vi "LSMcontroller_v56_from here for labview64bit.vi"() -> ()   [LabVIEW 2015] (continued)
                n3094 = property on="square matrix" class="Bool (strict)"("Value"=TRUE ("square matrix")) -> ()  [unwired: 2 in, 2 out]
                n3095 = property on="Square pixels" class="Bool (strict)"("Value"=FALSE ("square matrix")) -> ()  [unwired: 2 in, 2 out]
              }
            }
          }
          event "up", "downright", "down", "downleft", "right", "left", "upright", "upleft": Value Change {
            n3096 = event-data() -> ()  [unwired: 1 in, 6 out]
            n3097 = local read "downright"() -> (w6201:bool)
            n3098 = local read "downleft"() -> (w6203:bool)
            n3099 = local read "upright"() -> (w6199:bool)
            n3100 = local read "upleft"() -> (w6197:bool)
            n3101 = local read "down"() -> (w6202:bool)
            n3102 = local read "right"() -> (w6200:bool)
            n3103 = local read "left"() -> (w6204:bool)
            n3104 = local read "up"() -> (w6198:bool)
            n3105 = Compound Arithmetic op=OR(w6197, w6198, w6199, w6200, w6201, w6202, w6203, w6204) -> (w6196:bool)
            n3106 = case shown="True" w6196 {
              frame False {
              }
              frame True {
                n3107 = stacked-sequence {
                  frame #0 {
                    n3108 = local read "downright"() -> (w6206:bool)
                    n3109 = local read "downleft"() -> (w6208:bool)
                    n3110 = local read "BigSmall"() -> (w6205:bool)
                    n3111 = local read "upright"() -> (w6210:bool)
                    n3112 = local read "upleft"() -> (w6213:bool)
                    n3113 = local read "down"() -> (w6209:bool)
                    n3114 = local read "right"() -> (w6211:bool)
                    n3115 = local read "left"() -> (w6207:bool)
                    n3116 = local read "up"() -> (w6212:bool)
                    n3117 = call "movestageparams.vi"("command"="get") -> ("Params out"=w6216:T22)  [unwired: 1 in]
                    n3118 = Bundle By Name(cluster=w6216, "upleft"=w6213, "up"=w6212, "upright"=w6210, "right"=w6211, "downright"=w6206, "down"=w6209, "downleft"=w6208, "left"=w6207, "Bigsmall"=w6205) -> (w6217:T22)
                    n3119 = call "movestageparams.vi"("Params in"=w6217, "command"="set") -> ()  [unwired: 1 out]
                  }
                  frame #1 {
                    n3120 = disable-structure shown="Disabled" {
                      frame Disabled {
                        n3121 = call "configuration.vi"("command"="get") -> ("config out"=w6220:T13)  [unwired: 2 in, 1 out]
                        n3122 = in-place {
                          n3123 = in-place-cluster #45(w6220) -> ()  [unwired: 2 out]
                          n3124 = in-place-cluster #45("StageL"="StageL", "StageS"="StageS") -> (w6218:T13)
                        }
                        n3125 = call "configuration.vi"("config in"=w6218, "command"="set") -> ()  [unwired: 1 in, 2 out]
                      }
                      frame Enabled {
                      }
                    }
                  }
                  frame #2 {
                    n3126 = call "movestage.vi"() -> ()  [unwired: 12 in]
                  }
                  frame #3 {
                    w6224 = FALSE ("OK Button")
                    w6225 = FALSE ("OK Button")
                    n3127 = property on="down" class="Bool (strict)"("Value"=w6225) -> ()  [unwired: 2 in, 2 out]
                    n3128 = property on="up" class="Bool (strict)"("Value"=w6225) -> ()  [unwired: 2 in, 2 out]
                    n3129 = property on="right" class="Bool (strict)"("Value"=w6225) -> ()  [unwired: 2 in, 2 out]
                    n3130 = property on="left" class="Bool (strict)"("Value"=w6225) -> ()  [unwired: 2 in, 2 out]
                    n3131 = property on="upright" class="Bool (strict)"("Value"=w6224) -> ()  [unwired: 2 in, 2 out]
                    n3132 = property on="downleft" class="Bool (strict)"("Value"=w6224) -> ()  [unwired: 2 in, 2 out]
                    n3133 = property on="downright" class="Bool (strict)"("Value"=w6224) -> ()  [unwired: 2 in, 2 out]
                    n3134 = property on="upleft" class="Bool (strict)"("Value"=w6224) -> ()  [unwired: 2 in, 2 out]
                  }
                }
              }
            }
          }
          event "finite samples": Value Change {
            n3135 = event-data() -> ("NewVal"=w6226:bool)  [unwired: 1 in]
            n3136 = flat-sequence {
              tunnel: w6226 -> [w6227]
              frame #0 {
                n3137 = case shown="True" w6227 {
                  frame False {
                    w6228 = FALSE ("wavdet")
                    n3138 = property on="continuous" class="Bool (strict)"("Value"=TRUE ("continuous for display")) -> ()  [unwired: 2 in, 2 out]
                    n3139 = property on="wavdet" class="Bool (strict)"("Value"=w6228) -> ()  [unwired: 2 in, 2 out]
                    n3140 = property on="save\ndata" class="Bool (strict)"("Value"=w6228) -> ()  [unwired: 2 in, 2 out]
                    n3141 = property on="# of frames" class="DigNum (strict)"("DisabledEnum"=T8."Disabled and Grayed Out" ("Disabled")) -> ()  [unwired: 2 in, 2 out]
                    n3142 = property on="save\ndata" class="Bool (strict)"("DisabledEnum"=T8."Disabled and Grayed Out" ("Disabled")) -> ()  [unwired: 2 in, 2 out]
                    "Save tab" <- enum32{"withsave", "withoutsave"}."withsave" ("Save tab")
                  }
                  frame True {
                    w6235 = FALSE ("continuous for display")
                    n3143 = property on="continuous" class="Bool (strict)"("Value"=w6235) -> ()  [unwired: 2 in, 2 out]
                    n3144 = property on="wavdet" class="Bool (strict)"("Value"=w6235) -> ()  [unwired: 2 in, 2 out]
                    n3145 = local write "Save tab"(enum32{"withsave", "withoutsave"}."withsave" ("Save tab")) -> ()
                    n3146 = property on="save\ndata" class="Bool (strict)"("DisabledEnum"=T8."Enabled" ("Disabled")) -> ()  [unwired: 2 in, 2 out]
                    n3147 = property on="save\ndata" class="Bool (strict)"("Value"=TRUE ("save\ndata")) -> ()  [unwired: 2 in, 2 out]
                    n3148 = property on="# of frames" class="DigNum (strict)"("DisabledEnum"=T8."Enabled" ("Disabled")) -> ()  [unwired: 2 in, 2 out]
                  }
                }
              }
              frame #1 {
                n3149 = local read "finite samples"() -> (w6244:bool)
                n3150 = local read "continuous"() -> (w6243:bool)
                n3151 = local read "wavdet"() -> (w6242:bool)
                n3152 = call "2pparameters.vi"("command"="get") -> ("params out"=w6238:T12)  [unwired: 1 in]
                n3153 = Bundle By Name(cluster=w6238, "finite"=w6244, "cont"=w6243, "wavdet"=w6242) -> (w6241:T12)
                n3154 = call "2pparameters.vi"("Params in"=w6241, "command"="set") -> ()  [unwired: 1 out]
              }
            }
          }
          event "continuous": Value Change {
            n3155 = event-data() -> ("NewVal"=w6245:bool)  [unwired: 1 in]
            n3156 = flat-sequence {
              tunnel: w6245 -> [w6246]
              frame #0 {
                n3157 = case shown="True" w6246 {
                  frame False {
                    n3158 = property on="finite samples" class="Bool (strict)"("Value"=TRUE ("finite samples for recording")) -> ()  [unwired: 2 in, 2 out]
                    n3159 = property on="save\ndata" class="Bool (strict)"("Value"=TRUE ("save\ndata")) -> ()  [unwired: 2 in, 2 out]
                    n3160 = property on="wavdet" class="Bool (strict)"("Value"=FALSE ("wavdet")) -> ()  [unwired: 2 in, 2 out]
                    n3161 = local write "Save tab"(enum32{"withsave", "withoutsave"}."withsave" ("Save tab")) -> ()
                    n3162 = property on="# of frames" class="DigNum (strict)"("DisabledEnum"=T8."Enabled" ("Disabled")) -> ()  [unwired: 2 in, 2 out]
                    n3163 = property on="save\ndata" class="Bool (strict)"("DisabledEnum"=T8."Enabled" ("Disabled")) -> ()  [unwired: 2 in, 2 out]
                  }
                  frame True {
                    w6253 = FALSE ("finite samples for recording")
                    n3164 = property on="finite samples" class="Bool (strict)"("Value"=w6253) -> ()  [unwired: 2 in, 2 out]
                    n3165 = property on="wavdet" class="Bool (strict)"("Value"=w6253) -> ()  [unwired: 2 in, 2 out]
                    n3166 = property on="save\ndata" class="Bool (strict)"("Value"=w6253) -> ()  [unwired: 2 in, 2 out]
                    n3167 = local write "Save tab"(enum32{"withsave", "withoutsave"}."withsave" ("Save tab")) -> ()
                    n3168 = property on="# of frames" class="DigNum (strict)"("DisabledEnum"=T8."Disabled and Grayed Out" ("Disabled")) -> ()  [unwired: 2 in, 2 out]
                    n3169 = property on="save\ndata" class="Bool (strict)"("DisabledEnum"=T8."Disabled and Grayed Out" ("Disabled")) -> ()  [unwired: 2 in, 2 out]
                  }
                }
              }
              frame #1 {
                n3170 = local read "finite samples"() -> (w6263:bool)
                n3171 = local read "continuous"() -> (w6262:bool)
                n3172 = local read "wavdet"() -> (w6261:bool)
                n3173 = call "2pparameters.vi"("command"="get") -> ("params out"=w6257:T12)  [unwired: 1 in]
                n3174 = Bundle By Name(cluster=w6257, "finite"=w6263, "cont"=w6262, "wavdet"=w6261) -> (w6260:T12)
                n3175 = call "2pparameters.vi"("Params in"=w6260, "command"="set") -> ()  [unwired: 1 out]
              }
            }
          }
          event "wavdet": Value Change {
            n3176 = event-data() -> ("NewVal"=w6264:bool)  [unwired: 1 in]
            n3177 = flat-sequence {
              tunnel: w6264 -> [w6265]
              frame #0 {
                n3178 = case shown="False" w6265 {
                  frame False {
                    n3179 = property on="finite samples" class="Bool (strict)"("Value"=TRUE ("finite samples for recording")) -> ()  [unwired: 2 in, 2 out]
                    n3180 = property on="continuous" class="Bool (strict)"("Value"=FALSE ("continuous")) -> ()  [unwired: 2 in, 2 out]
                    n3181 = local write "Save tab"(enum32{"withsave", "withoutsave"}."withsave" ("Save tab")) -> ()
                    n3182 = property on="save\ndata" class="Bool (strict)"("DisabledEnum"=T8."Enabled" ("Disabled")) -> ()  [unwired: 2 in, 2 out]
                    n3183 = property on="# of frames" class="DigNum (strict)"("DisabledEnum"=T8."Enabled" ("Disabled")) -> ()  [unwired: 2 in, 2 out]
                    n3184 = property on="save\ndata" class="Bool (strict)"("Value"=TRUE ("save\ndata")) -> ()  [unwired: 2 in, 2 out]
                  }
                  frame True {
                    w6274 = FALSE ("finite samples for recording")
                    n3185 = property on="finite samples" class="Bool (strict)"("Value"=w6274) -> ()  [unwired: 2 in, 2 out]
                    n3186 = property on="continuous" class="Bool (strict)"("Value"=w6274) -> ()  [unwired: 2 in, 2 out]
                    n3187 = property on="save\ndata" class="Bool (strict)"("DisabledEnum"=T8."Enabled" ("Disabled")) -> ()  [unwired: 2 in, 2 out]
                    n3188 = local write "Save tab"(enum32{"withsave", "withoutsave"}."withsave" ("Save tab")) -> ()
                    n3189 = property on="# of frames" class="DigNum (strict)"("DisabledEnum"=T8."Disabled" ("Disabled")) -> ()  [unwired: 2 in, 2 out]
                    n3190 = property on="save\ndata" class="Bool (strict)"("Value"=TRUE ("save\ndata")) -> ()  [unwired: 2 in, 2 out]
                  }
                }
              }
              frame #1 {
                n3191 = local read "finite samples"() -> (w6277:bool)
                n3192 = local read "continuous"() -> (w6278:bool)
                n3193 = local read "wavdet"() -> (w6279:bool)
                n3194 = call "2pparameters.vi"("command"="get") -> ("params out"=w6283:T12)  [unwired: 1 in]
                n3195 = Bundle By Name(cluster=w6283, "finite"=w6277, "cont"=w6278, "wavdet"=w6279) -> (w6280:T12)
                n3196 = call "2pparameters.vi"("Params in"=w6280, "command"="set") -> ()  [unwired: 1 out]
              }
            }
          }
          event "cursors": Value Change {
            n3197 = event-data() -> ()  [unwired: 1 in, 5 out]
            n3198 = case shown="True" "cursors" {
              frame False {
                n3199 = property on="img_CH1" class="IntGraph (strict)"("Active Cursor"=u32 0, "Cursor.Cursor Style"=u8 0 ("Cursor Style"), "Cursor.Cursor Point Style"=u8 0 ("Cursor Point Style")) -> ("Cursor.Cursor Position:Cursor X"=w6288:dbl, "Cursor.Cursor Position:Cursor Y"=w6289:dbl)  [unwired: 2 in, 2 out]
                n3200 = property on="img_CH2" class="IntGraph (strict)"("Active Cursor"=u32 0, "Cursor.Cursor Style"=u8 0 ("Cursor Style"), "Cursor.Cursor Point Style"=u8 0 ("Cursor Point Style")) -> ()  [unwired: 2 in, 2 out]
                n3201 = local write "cursor x [pixel]"(w6288) -> ()
                n3202 = local write "cursor y [pixel]"(w6289) -> ()
              }
              frame True {
                n3203 = stacked-sequence {
                  frame #0 {
                    n3204 = call "2pparameters.vi"("command"="get") -> ("params out"=w6304:T12)  [unwired: 1 in]
                    n3205 = Unbundle By Name(w6304) -> ("Xpixels Img"=w6305:i32, "Ypixels Img"=w6302:i32)
                    n3206 = To Double Precision Float(number=w6302) -> (double precision float=w6296:dbl)
                    n3207 = To Double Precision Float(number=w6305) -> (double precision float=w6301:dbl)
                    n3208 = Divide(x=w6296, y=2.0) -> (x/y=w6297:dbl)
                    n3209 = Divide(x=w6301, y=2.0) -> (x/y=w6299:dbl)
                    n3210 = Round To Nearest(number=w6297) -> (nearest integer value=w6295:dbl)
                    n3211 = Round To Nearest(number=w6299) -> (nearest integer value=w6298:dbl)
                    n3212 = property on="img_CH1" class="IntGraph (strict)"("Active Cursor"=u32 0, "Cursor.Cursor Style"=u8 8 ("Cursor Style"), "Cursor.Cursor Point Style"=u8 5 ("Cursor Point Style"), "Cursor.Cursor Position:Cursor X"=w6298, "Cursor.Cursor Position:Cursor Y"=w6295, "Cursor.Visible"=TRUE) -> ()  [unwired: 2 in, 2 out]
                  }
                  frame #1 {
                    n3213 = call "2pparameters.vi"("command"="get") -> ("params out"=w6324:T12)  [unwired: 1 in]
                    n3214 = call "2pparameters.vi"("command"="get") -> ("params out"=w6322:T12)  [unwired: 1 in]
                    n3215 = property on="img_CH1" class="IntGraph (strict)"("Active Cursor"=u32 0, "Cursor.Cursor Style"=u8 8 ("Cursor Style"), "Cursor.Cursor Point Style"=u8 5 ("Cursor Point Style")) -> ("Cursor.Cursor Position:Cursor X"=w6317:dbl, "Cursor.Cursor Position:Cursor Y"=w6316:dbl, "Cursor.Cursor Index"=w6339:i32, "Cursor.Cursor Plot"=w6338:i32, "Cursor.Visible"=w6309:bool)  [unwired: 2 in, 2 out]
                    "cursor x [pixel]" <- w6317
                    "cursor y [pixel]" <- w6316
                    n3216 = Unbundle By Name(w6324) -> ("Vy-max Img"=w6326:dbl, "Vy-min Img"=w6313:dbl, "Ypixels Img"=w6328:i32)
                    n3217 = Unbundle By Name(w6322) -> ("VX-max Img"=w6323:dbl, "Vx-min Img"=w6311:dbl, "Xpixels Img"=w6327:i32)
                    n3218 = Subtract(x=w6326, y=w6313) -> (x-y=w6331:dbl)
                    n3219 = Subtract(x=w6323, y=w6311) -> (x-y=w6329:dbl)
                    n3220 = local read "img_CH2"() -> (w6335:sgl[][])
                    n3221 = To Double Precision Float(number=w6327) -> (double precision float=w6330:dbl)
                    n3222 = local read "img_CH1"() -> (w6336:sgl[][])
                    n3223 = To Double Precision Float(number=w6328) -> (double precision float=w6332:dbl)
                    n3224 = Index Array(array=w6336, index (row)=w6339, index (col)=w6338) -> (element=→"value CH 1":sgl)
                    n3225 = Index Array(array=w6335, index (row)=w6339, index (col)=w6338) -> (element=→"value CH 2":sgl)
                    n3226 = Divide(x=w6329, y=w6330) -> (x/y=w6333:dbl)
                    n3227 = Divide(x=w6331, y=w6332) -> (x/y=w6334:dbl)
                    n3228 = Multiply(x=w6317, y=w6333) -> (x*y=w6312:dbl)
                    n3229 = Multiply(x=w6316, y=w6334) -> (x*y=w6315:dbl)
                    n3230 = property on="img_CH2" class="IntGraph (strict)"("Active Cursor"=u32 0, "Cursor.Cursor Style"=u8 8 ("Cursor Style"), "Cursor.Cursor Point Style"=u8 5 ("Cursor Point Style"), "Cursor.Cursor Position:Cursor X"=w6317, "Cursor.Cursor Position:Cursor Y"=w6316, "Cursor.Visible"=w6309) -> ()  [unwired: 2 in, 2 out]
                    n3231 = Add(x=w6312, y=w6311) -> (x+y=w6310:dbl)
                    n3232 = Add(x=w6315, y=w6313) -> (x+y=w6314:dbl)
                    n3233 = local write "Vx-ref"(w6310) -> ()
                    n3234 = local write "Vy-ref"(w6314) -> ()
                  }
                }
              }
            }
          }
          event "img_CH1": Cursor Move {
            n3235 = event-data() -> ("CursIdx"=w6344:i32)  [unwired: 1 in]
            n3236 = Equal To 0?(x=w6344) -> (x = 0?=w6345:bool)
            n3237 = case shown="True" w6345 {
              frame False {
              }
              frame True {
                n3238 = call "2pparameters.vi"("command"="get") -> ("params out"=w6365:T12)  [unwired: 1 in]
                n3239 = call "2pparameters.vi"("command"="get") -> ("params out"=w6367:T12)  [unwired: 1 in]
                n3240 = property on="img_CH1" class="IntGraph (strict)"("Active Cursor"=u32 0, "Cursor.Cursor Style"=u8 8 ("Cursor Style"), "Cursor.Cursor Point Style"=u8 5 ("Cursor Point Style")) -> ("Cursor.Cursor Position:Cursor X"=w6354:dbl, "Cursor.Cursor Position:Cursor Y"=w6353:dbl, "Cursor.Cursor Plot"=w6373:i32, "Cursor.Cursor Index"=w6372:i32, "Cursor.Visible"=w6346:bool)  [unwired: 2 in, 2 out]
                n3241 = Unbundle By Name(w6365) -> ("Vy-max Img"=w6363:dbl, "Vy-min Img"=w6352:dbl, "Ypixels Img"=w6361:i32)
                n3242 = Unbundle By Name(w6367) -> ("VX-max Img"=w6366:dbl, "Vx-min Img"=w6347:dbl, "Xpixels Img"=w6362:i32)
                n3243 = Subtract(x=w6363, y=w6352) -> (x-y=w6358:dbl)
                n3244 = Subtract(x=w6366, y=w6347) -> (x-y=w6360:dbl)
                n3245 = local write "cursor x [pixel]"(w6354) -> ()
                n3246 = local write "cursor y [pixel]"(w6353) -> ()
                n3247 = To Double Precision Float(number=w6362) -> (double precision float=w6359:dbl)
                n3248 = To Double Precision Float(number=w6361) -> (double precision float=w6357:dbl)
                n3249 = local read "img_CH2"() -> (w6374:sgl[][])
                n3250 = local read "img_CH1"() -> (w6377:sgl[][])
                n3251 = Index Array(array=w6374, index (row)=w6373, index (col)=w6372) -> (element=w6375:sgl)
                n3252 = Index Array(array=w6377, index (row)=w6373, index (col)=w6372) -> (element=w6376:sgl)
                n3253 = Divide(x=w6360, y=w6359) -> (x/y=w6356:dbl)
                n3254 = Divide(x=w6358, y=w6357) -> (x/y=w6355:dbl)
                n3255 = local write "value CH 2"(w6375) -> ()
                n3256 = Multiply(x=w6354, y=w6356) -> (x*y=w6349:dbl)
                n3257 = local write "value CH 1"(w6376) -> ()
                n3258 = Multiply(x=w6353, y=w6355) -> (x*y=w6351:dbl)
                n3259 = Add(x=w6349, y=w6347) -> (x+y=w6348:dbl)
                n3260 = local write "Vx-ref"(w6348) -> ()
                n3261 = Add(x=w6351, y=w6352) -> (x+y=w6350:dbl)
                n3262 = property on="img_CH2" class="IntGraph (strict)"("Active Cursor"=u32 0, "Cursor.Cursor Style"=u8 8 ("Cursor Style"), "Cursor.Cursor Point Style"=u8 5 ("Cursor Point Style"), "Cursor.Cursor Position:Cursor X"=w6354, "Cursor.Cursor Position:Cursor Y"=w6353, "Cursor.Visible"=w6346) -> ()  [unwired: 2 in, 2 out]
                n3263 = local write "Vy-ref"(w6350) -> ()
              }
            }
          }
          event "img_CH2": Cursor Move {
            n3264 = event-data() -> ("CursIdx"=w6381:i32)  [unwired: 1 in]
            n3265 = Equal To 0?(x=w6381) -> (x = 0?=w6382:bool)
            n3266 = case shown="True" w6382 {
              frame False {
              }
              frame True {
                n3267 = property on="img_CH2" class="IntGraph (strict)"("Active Cursor"=u32 0, "Cursor.Cursor Style"=u8 8 ("Cursor Style"), "Cursor.Cursor Point Style"=u8 5 ("Cursor Point Style")) -> ("Cursor.Cursor Position:Cursor X"=w6390:dbl, "Cursor.Cursor Position:Cursor Y"=w6391:dbl, "Cursor.Cursor Plot"=w6410:i32, "Cursor.Cursor Index"=w6409:i32, "Cursor.Visible"=w6383:bool)  [unwired: 2 in, 2 out]
                n3268 = call "2pparameters.vi"("command"="get") -> ("params out"=w6402:T12)  [unwired: 1 in]
                n3269 = call "2pparameters.vi"("command"="get") -> ("params out"=w6404:T12)  [unwired: 1 in]
                n3270 = local read "img_CH1"() -> (w6414:sgl[][])
                n3271 = local read "img_CH2"() -> (w6411:sgl[][])
                n3272 = local write "cursor x [pixel]"(w6390) -> ()
                n3273 = local write "cursor y [pixel]"(w6391) -> ()
                n3274 = Unbundle By Name(w6402) -> ("Vy-max Img"=w6400:dbl, "Vy-min Img"=w6385:dbl, "Ypixels Img"=w6398:i32)
                n3275 = Unbundle By Name(w6404) -> ("VX-max Img"=w6403:dbl, "Vx-min Img"=w6388:dbl, "Xpixels Img"=w6399:i32)
                n3276 = Index Array(array=w6414, index (row)=w6410, index (col)=w6409) -> (element=w6413:sgl)
                n3277 = Index Array(array=w6411, index (row)=w6410, index (col)=w6409) -> (element=w6412:sgl)
                n3278 = local write "value CH 2"(w6412) -> ()
                n3279 = local write "value CH 1"(w6413) -> ()
                n3280 = Subtract(x=w6400, y=w6385) -> (x-y=w6395:dbl)
                n3281 = Subtract(x=w6403, y=w6388) -> (x-y=w6397:dbl)
                n3282 = To Double Precision Float(number=w6399) -> (double precision float=w6396:dbl)
                n3283 = To Double Precision Float(number=w6398) -> (double precision float=w6394:dbl)
                n3284 = Divide(x=w6397, y=w6396) -> (x/y=w6393:dbl)
                n3285 = Divide(x=w6395, y=w6394) -> (x/y=w6392:dbl)
                n3286 = Multiply(x=w6390, y=w6393) -> (x*y=w6389:dbl)
                n3287 = Multiply(x=w6391, y=w6392) -> (x*y=w6386:dbl)
                n3288 = property on="img_CH1" class="IntGraph (strict)"("Active Cursor"=u32 0, "Cursor.Cursor Style"=u8 8 ("Cursor Style"), "Cursor.Cursor Point Style"=u8 5 ("Cursor Point Style"), "Cursor.Cursor Position:Cursor X"=w6390, "Cursor.Cursor Position:Cursor Y"=w6391, "Cursor.Visible"=w6383) -> ()  [unwired: 2 in, 2 out]
                n3289 = Add(x=w6389, y=w6388) -> (x+y=→"Vx-ref":dbl)
                n3290 = Add(x=w6386, y=w6385) -> (x+y=→"Vy-ref":dbl)
              }
            }
          }
          event "auto shutter": Value Change {
            n3291 = event-data() -> ()  [unwired: 1 in, 6 out]
            n3292 = call "2pparameters.vi"("command"="get") -> ("params out"=w6420:T12)  [unwired: 1 in]
            n3293 = in-place {
              n3294 = in-place-cluster #46(w6420) -> ()  [unwired: 1 out]
              n3295 = local read "auto shutter"() -> (w6422:bool)
              n3296 = in-place-cluster #46("autoshutter"=w6422) -> (w6418:T12)
            }
            n3297 = call "2pparameters.vi"("Params in"=w6418, "command"="set") -> ()  [unwired: 1 out]
          }
          event "auto OD": Value Change {
            n3298 = event-data() -> ()  [unwired: 1 in, 6 out]
            n3299 = call "2pparameters.vi"("command"="get") -> ("params out"=w6425:T12)  [unwired: 1 in]
            n3300 = in-place {
              n3301 = in-place-cluster #47(w6425) -> ()  [unwired: 1 out]
              n3302 = local read "auto OD"() -> (w6427:bool)
              n3303 = in-place-cluster #47("auto OD"=w6427) -> (w6423:T12)
            }
            n3304 = call "2pparameters.vi"("Params in"=w6423, "command"="set") -> ()  [unwired: 1 out]
          }
          event "ODfilt": Value Change {
            n3305 = event-data() -> ("OldVal"=w6428:u16)  [unwired: 1 in, 5 out]
            n3306 = local read "ODfilt"() -> (w6429:u16)
            n3307 = call "2pparameters.vi"("command"="get") -> ("params out"=w6432:T12)  [unwired: 1 in]
            n3308 = call "filterwheelcontrol_nothorlabslib.vi"("Current OD filt"=w6428, "New ODfilt"=w6429) -> ()  [unwired: 1 in]
            n3309 = in-place {
              in-place-border: w6429 -> [w6434]
              n3310 = in-place-cluster #48(w6432) -> ()  [unwired: 1 out]
              n3311 = in-place-cluster #48("ODfilt"=w6434) -> (w6430:T12)
            }
            n3312 = call "2pparameters.vi"("Params in"=w6430, "command"="set") -> ()  [unwired: 1 out]
          }
          event "Exit": Value Change {
            n3313 = event-data() -> ()  [unwired: 1 in, 5 out]
          }
        }
        n3314 = Wait (ms)(milliseconds to wait=u32 50) -> ()  [unwired: 1 out]
      }
      n3315 = while {
        stop <- w75 stop-if-true
        # "Waveform generation"
        n3316 = event shown="[1] \"Add AO wave\": Value Change" {
          selector: _ -> [_ _ _ _ _ _ _ _ _ _ _ _ _ _ _ _ _]
          dyn-events: _ -> [_ _ _ _ _ _ _ _ _ _ _ _ _ _ _ _ _]
          timeout: _ -> [_ _ _ _ _ _ _ _ _ _ _ _ _ _ _ _ _]
          tunnel: [_ _ _ _ _ _ _ _ _ _ _ _ _ _ _ _ w2048] -> w75
          event Timeout {
            n3317 = event-data() -> ()  [unwired: 1 in, 3 out]
          }
          event "Add AO wave": Value Change {
            n3318 = event-data() -> ("NewVal"=w76:bool)  [unwired: 1 in, 5 out]
            n3319 = case shown="True" w76 {
              frame False {
              }
              frame True {
                n3320 = stacked-sequence {
                  frame #0 {
                    n3321 = local read "Measurement"() -> (w77:T5)
                    n3322 = case shown="\"Lifetime (contour)\"" w77 {
                      frame "X-Y-t movie", Default {
                        n3323 = local read "avpp"() -> (w98:i32)
                        n3324 = local read "Angle ref"() -> (w97:dbl)
                        n3325 = local read "ROI Type"() -> (w96:u16)
                        n3326 = local read "xpixels ref"() -> (w93:i32)
                        n3327 = local read "Vx-min ref"() -> (w92:dbl)
                        n3328 = local read "Vx-max ref"() -> (w91:dbl)
                        n3329 = local read "ypixels ref"() -> (w89:i32)
                        n3330 = local read "Vy-min ref"() -> (w90:dbl)
                        n3331 = local read "Vy-max ref"() -> (w86:dbl)
                        n3332 = local read "Sampling rate"() -> (w80:dbl)
                        n3333 = local read "finite samples"() -> (w81:bool)
                        n3334 = local read "continuous"() -> (w84:bool)
                        n3335 = local read "wavdet"() -> (w85:bool)
                        n3336 = local read "# of frames"() -> (w83:i32)
                        n3337 = local read "maxbufferAI"() -> (w82:i32)
                        n3338 = local read "Override AI buffer"() -> (w78:bool)
                        n3339 = call "2pparameters.vi"("command"="get") -> ("params out"=w95:T12)  [unwired: 1 in]
                        n3340 = Bundle By Name(cluster=w95, "type"="X-Y-t movie", "avpp"=w98, "Angle Img"=w97, "Xpixels Img"=w93, "Vx-min Img"=w92, "VX-max Img"=w91, "Ypixels Img"=w89, "Vy-min Img"=w90, "Vy-max Img"=w86, "srate"=w80, "srate Img"=w80, "finite"=w81, "cont"=w84, "wavdet"=w85, "measpoints"=w83, "maxbufferAI"=w82, "Drawing Mode"=w96, "Vz-reset"=0.0, "AIoverride"=w78) -> (w87:T12)
                        n3341 = call "2pparameters.vi"("Params in"=w87, "command"="set") -> ()  [unwired: 1 out]
                      }
                      frame "X-Y-Z stack" {
                        n3342 = call "2pparameters.vi"("command"="get") -> ("params out"=w102:T12)  [unwired: 1 in]
                        n3343 = Bundle By Name(cluster=w102, "type"="X-Y-Z stack") -> (w100:T12)
                        n3344 = call "2pparameters.vi"("Params in"=w100, "command"="set") -> ()  [unwired: 1 out]
                      }
                      frame "Lifetime (scan)" {
                        n3345 = call "2pparameters.vi"("command"="get") -> ("params out"=w107:T12)  [unwired: 1 in]
                        n3346 = Bundle By Name(cluster=w107, "type"="Lifetime (scan)") -> (w105:T12)
                        n3347 = call "2pparameters.vi"("Params in"=w105, "command"="set") -> ()  [unwired: 1 out]
                      }
                      frame "Lifetime (contour)" {
                        n3348 = local read "Vy-min draw"() -> (w117:dbl)
                        n3349 = local read "Vy-max draw"() -> (w116:dbl)
                        n3350 = local read "Vx-min draw"() -> (w119:dbl)
                        n3351 = local read "Vx-max draw"() -> (w118:dbl)
                        n3352 = local read "xpixels ref"() -> (w115:i32)
                        n3353 = local read "ypixels ref"() -> (w114:i32)
                        n3354 = local read "ROI Type"() -> (w113:u16)
                        n3355 = local read "srateAODOtt"() -> (w124:dbl)
                        n3356 = local read "# of frames"() -> (w129:i32)
                        n3357 = local read "refreshtime"() -> (w121:dbl)
                        n3358 = local read "Pel"() -> (w112:dbl)
                        n3359 = local read "bin"() -> (w127:dbl)
                        n3360 = local read "Override AI buffer"() -> (w110:bool)
                        n3361 = local read "finite samples"() -> (w136:bool)
                        n3362 = local read "srateAODOtt"() -> (w123:dbl)
                        n3363 = local read "srateAODOtt"() -> (w130:dbl)
                        n3364 = local read "continuous"() -> (w135:bool)
                        n3365 = local read "Angle ref"() -> (w120:dbl)
                        n3366 = local read "wavdet"() -> (w137:bool)
                        n3367 = local read "Vx-ref"() -> (w132:dbl)
                        n3368 = local read "Vy-ref"() -> (w134:dbl)
                        n3369 = local read "avpp"() -> (w133:i32)
                        n3370 = call "tt_timeandsamples.vi"("bin"=w127, "refreshtime"=w121, "srateAODOtt"=w124, "tot#ofsamples"=w129) -> ("refreshrate"=w125:dbl, "refreshbuffer"=w126:i32, "timetracecycles"=w131:i32)  [unwired: 5 in]
                        n3371 = local read "bin"() -> (w128:dbl)
                        n3372 = call "2pparameters.vi"("command"="get") -> ("params out"=w140:T12)  [unwired: 1 in]
                        n3373 = Bundle By Name(cluster=w140, "Drawing Mode"=w113, "measpoints"=w129, "tt_cycles"=w131, "refreshbuffer"=w126, "refreshrate"=w125, "Vx-ref"=w132, "Vy-ref"=w134, "srate"=w123, "finite"=w136, "cont"=w135, "wavdet"=w137, "avpp"=w133, "srateAODO"=w130, "bufferAI"=w126, "bin"=w128, "Angle Img"=w120, "Vxminref"=w119, "Vxmaxref"=w118, "Vyminref"=w117, "Vymaxref"=w116, "Xpixels Img"=w115, "Ypixels Img"=w114, "Pel"=w112, "Vz-reset"=0.0, "AIoverride"=w110, "type"="Lifetime (contour)") -> (w138:T12)
                        n3374 = Reciprocal(x=w125) -> (1/x=w122:dbl)
                        n3375 = local write "refreshtime"(w122) -> ()
                        n3376 = call "2pparameters.vi"("Params in"=w138, "command"="set") -> ()  [unwired: 1 out]
                      }
                      frame "X-Y-Z-t movie" {
                      }
                      frame "linescan" {
                      }
                      frame "Timetrace" {
                        n3377 = local read "Vy-min draw"() -> (w150:dbl)
                        n3378 = local read "Vy-max draw"() -> (w149:dbl)
                        n3379 = local read "Vx-min draw"() -> (w152:dbl)
                        n3380 = local read "Vx-max draw"() -> (w151:dbl)
                        n3381 = local read "xpixels ref"() -> (w148:i32)
                        n3382 = local read "ypixels ref"() -> (w147:i32)
                        n3383 = local read "ROI Type"() -> (w146:u16)
                        n3384 = local read "srateAODOtt"() -> (w157:dbl)
                        n3385 = local read "# of frames"() -> (w162:i32)
                        n3386 = local read "refreshtime"() -> (w154:dbl)
                        n3387 = local read "Pel"() -> (w145:dbl)
                        n3388 = local read "bin"() -> (w160:dbl)
                        n3389 = local read "Override AI buffer"() -> (w143:bool)
                        n3390 = local read "finite samples"() -> (w169:bool)
                        n3391 = local read "srateAODOtt"() -> (w156:dbl)
                        n3392 = local read "srateAODOtt"() -> (w163:dbl)
                        n3393 = local read "continuous"() -> (w168:bool)
                        n3394 = local read "Angle ref"() -> (w153:dbl)
                        n3395 = local read "wavdet"() -> (w170:bool)
                        n3396 = local read "Vx-ref"() -> (w165:dbl)
                        n3397 = local read "Vy-ref"() -> (w167:dbl)
                        n3398 = local read "avpp"() -> (w166:i32)
                        n3399 = call "tt_timeandsamples.vi"("bin"=w160, "refreshtime"=w154, "srateAODOtt"=w157, "tot#ofsamples"=w162) -> ("refreshrate"=w158:dbl, "refreshbuffer"=w159:i32, "timetracecycles"=w164:i32)  [unwired: 5 in]
                        n3400 = local read "bin"() -> (w161:dbl)
                        n3401 = call "2pparameters.vi"("command"="get") -> ("params out"=w173:T12)  [unwired: 1 in]
                        n3402 = Bundle By Name(cluster=w173, "Drawing Mode"=w146, "measpoints"=w162, "tt_cycles"=w164, "refreshbuffer"=w159, "refreshrate"=w158, "Vx-ref"=w165, "Vy-ref"=w167, "srate"=w156, "finite"=w169, "cont"=w168, "wavdet"=w170, "avpp"=w166, "srateAODO"=w163, "bufferAI"=w159, "bin"=w161, "Angle Img"=w153, "Vxminref"=w152, "Vxmaxref"=w151, "Vyminref"=w150, "Vymaxref"=w149, "Xpixels Img"=w148, "Ypixels Img"=w147, "Pel"=w145, "Vz-reset"=0.0, "AIoverride"=w143, "type"="Timetrace") -> (w171:T12)
                        n3403 = Reciprocal(x=w158) -> (1/x=w155:dbl)
                        n3404 = local write "refreshtime"(w155) -> ()
                        n3405 = call "2pparameters.vi"("Params in"=w171, "command"="set") -> ()  [unwired: 1 out]
                      }
                      frame "Lifetime (point)" {
                      }
                    }
                  }
                  frame #1 {
                    w176 = FALSE ("wavdet")
                    n3406 = call "2pparameters.vi"("command"="get") -> ("params out"=w180:T12)  [unwired: 1 in]
                    n3407 = Bundle By Name(cluster=w180, "finite"=w176, "cont"=w176, "wavdet"=TRUE) -> (w177:T12)
                    n3408 = call "2pparameters.vi"("Params in"=w177, "command"="set") -> ()  [unwired: 1 out]
                  }
                  frame #2 {
                    # "change active waveform numbers array"
                    n3409 = local read "AO channels"() -> (w187:u32)
                    n3410 = call "2pparameters.vi"("command"="get") -> ("params out"=w185:T12)  [unwired: 1 in]
                    n3411 = in-place {
                      in-place-border: w187 -> [w191]
                      in-place-border: [w188] -> w182
                      n3412 = in-place-cluster #49(w185) -> ("aAO"=w190:u32[])
                      n3413 = call "add channel to active arrayv2.vi"("line array in"=w190, "line to add"=w191) -> ("line array out"=w189:u32[], "addition"=w188:bool)  [unwired: 1 out]
                      n3414 = in-place-cluster #49("aAO"=w189) -> (w183:T12)
                    }
                    n3415 = local write "addAO"(w182) -> ()
                    n3416 = call "2pparameters.vi"("Params in"=w183, "command"="set") -> ()  [unwired: 1 out]
                  }
                  frame #3 {
                    # "update GUI"
                    n3417 = local read "addAO"() -> (w192:bool)
                    n3418 = case shown="True" w192 {
                      frame False {
                      }
                      frame True {
                        n3419 = call "Used AO lines.vi"() -> ("used AO names"=w196:string[], "used AO lines"=w198:tag[])  [unwired: 2 in]
                        n3420 = control-ref of="Analog Lines Plot"() -> (w197:refnum<vi>)
                        n3421 = control-ref of="Digital Lines Plot"() -> (w195:refnum<vi>)
                        n3422 = call "Used DO lines.vi"() -> ("used DO names"=w194:string[], "used DO lines"=w193:tag[])  [unwired: 2 in]
                        n3423 = local write "Analog Used Lines"(w198) -> ()
                        n3424 = local write "Analog Used Names"(w196) -> ()
                        n3425 = local write "Digital Used Lines"(w193) -> ()
                        n3426 = local write "Digital Used Names"(w194) -> ()
                        n3427 = call "prepDOWaveplot.vi"("DigitalGraph in"=w195, "used DO names"=w194) -> ()  [unwired: 1 in]
                        n3428 = call "prepAOWaveplot.vi"("WaveformGraph in"=w197, "Analog Used Names"=w196) -> ()  [unwired: 1 in]
                      }
                    }
                  }
                  frame #4 {
                    n3429 = local read "addAO"() -> (w199:bool)
                    n3430 = case shown="True" w199 {
                      frame False {
                      }
                      frame True {
                        # "add parameters\nto parameter array"
                        n3431 = local read "Build analog waveform tabs"() -> (w200:enum32{"Square", "Triangle", "Matlab"})
                        n3432 = case shown="\"Square\", Default" w200 {
                          frame "Square", Default {
                            w213 = 0.0 ("Offset (V)")
                            n3433 = local read "Meastab"() -> (w202:enum32{"X-Y Image", "Linescan", "Timetrace"})
                            n3434 = call "waveformparamsv2.vi"("command"="get") -> ("Params out"=w211:T16)  [unwired: 4 in, 2 out]
                            n3435 = Unbundle By Name(w211) -> ("AO parameters"=w208:T17)
                            n3436 = case shown="\"Timetrace\"" w202 {
                              tunnel: [w224 w225] -> w201
                              frame "X-Y Image", Default {
                                n3437 = local read "Sampling rate"() -> (w224:dbl)
                              }
                              frame "Timetrace" {
                                n3438 = local read "srateAODOtt"() -> (w225:dbl)
                              }
                            }
                            n3439 = local read "Start amplitude (V)"() -> (w221:dbl)
                            n3440 = local read "phase shift (ms)"() -> (w214:dbl)
                            n3441 = local read "Step size (V)"() -> (w219:dbl)
                            n3442 = local read "Baseline (V)"() -> (w220:dbl)
                            n3443 = local read "Period (ms)"() -> (w217:dbl)
                            n3444 = local read "padding value"() -> (w204:dbl)
                            n3445 = local read "Repeats"() -> (w223:dbl)
                            n3446 = local read "DC (%)"() -> (w218:dbl)
                            n3447 = local read "Cycles"() -> (w222:dbl)
                            n3448 = local read "Pulses"() -> (w215:dbl)
                            n3449 = Index Array(array=w208, index=0) -> (element=w209:T18)
                            n3450 = Bundle By Name(cluster=w209, "AOtab"=0.0 ("Repeats"), "Repeats"=w223, "Cycles"=w222, "Start amplitude (V)"=w221, "Baseline (V)"=w220, "Step size (V)"=w219, "DC (%)"=w218, "Sampling frequency (Hz)"=w201, "Period (ms)"=w217, "Offset (V)"=w213, "Amplitude (V)"=w213, "Frequency"=w213, "Tri Repeats"=w213, "phase shift (ms)"=w214, "Pulses"=w215, "Matlab wave file"=path "", "padding value"=w204) -> (w206:T18)
                            n3451 = Build Array(w206) -> (w205:T17)
                            n3452 = call "waveformparamsv2.vi"("command"="add AO", "add AO"=w205) -> ()  [unwired: 3 in, 3 out]
                          }
                          frame "Matlab" {
                            w231 = 0.0 ("Repeats")
                            n3453 = local read "Meastab"() -> (w227:enum32{"X-Y Image", "Linescan", "Timetrace"})
                            n3454 = call "waveformparamsv2.vi"("command"="get") -> ("Params out"=w238:T16)  [unwired: 4 in, 2 out]
                            n3455 = Unbundle By Name(w238) -> ("AO parameters"=w235:T17)
                            n3456 = case shown="\"Timetrace\"" w227 {
                              tunnel: [w241 w242] -> w226
                              frame "X-Y Image", Default {
                                n3457 = local read "Sampling rate"() -> (w241:dbl)
                              }
                              frame "Timetrace" {
                                n3458 = local read "srateAODOtt"() -> (w242:dbl)
                              }
                            }
                            n3459 = local read "Matlab waveform path"() -> (w228:path)
                            n3460 = local read "Matlab padding value"() -> (w230:dbl)
                            n3461 = Index Array(array=w235, index=0) -> (element=w236:T18)
                            n3462 = call "matlabwfexistsdialogue.vi"("Matlab waveform path"=w228) -> ("mtalab waveform path out"=w229:path)
                            n3463 = Bundle By Name(cluster=w236, "AOtab"=2.0 ("Repeats"), "Repeats"=w231, "Cycles"=w231, "Start amplitude (V)"=w231, "Baseline (V)"=w231, "Step size (V)"=w231, "DC (%)"=w231, "Sampling frequency (Hz)"=w226, "Period (ms)"=w231, "Offset (V)"=w231, "Amplitude (V)"=w231, "Frequency"=w231, "Tri Repeats"=w231, "phase shift (ms)"=w231, "Pulses"=w231, "Matlab wave file"=w229, "padding value"=w230) -> (w233:T18)
                            n3464 = Build Array(w233) -> (w232:T17)
                            n3465 = call "waveformparamsv2.vi"("command"="add AO", "add AO"=w232) -> ()  [unwired: 3 in, 3 out]
                          }
                          frame "Triangle" {
                            w248 = 0.0 ("Offset (V)")
                            n3466 = local read "Meastab"() -> (w244:enum32{"X-Y Image", "Linescan", "Timetrace"})
                            n3467 = call "waveformparamsv2.vi"("command"="get") -> ("Params out"=w260:T16)  [unwired: 4 in, 2 out]
                            n3468 = Unbundle By Name(w260) -> ("AO parameters"=w257:T17)
                            n3469 = case shown="\"Timetrace\"" w244 {
                              tunnel: [w262 w263] -> w243
                              frame "X-Y Image", Default {
                                n3470 = local read "Sampling rate"() -> (w262:dbl)
                              }
                              frame "Timetrace" {
                                n3471 = local read "srateAODOtt"() -> (w263:dbl)
                              }
                            }
                            n3472 = local read "Tri padding value"() -> (w246:dbl)
                            n3473 = local read "Amplitude (V)"() -> (w251:dbl)
                            n3474 = local read "Tri Phase (s)"() -> (w247:dbl)
                            n3475 = local read "Tri Repeats"() -> (w249:dbl)
                            n3476 = local read "Frequency"() -> (w250:dbl)
                            n3477 = local read "Offset (V)"() -> (w252:dbl)
                            n3478 = Index Array(array=w257, index=0) -> (element=w258:T18)
                            n3479 = Bundle By Name(cluster=w258, "AOtab"=1.0 ("Repeats"), "Repeats"=w248, "Cycles"=w248, "Start amplitude (V)"=w248, "Baseline (V)"=w248, "Step size (V)"=w248, "DC (%)"=w248, "Sampling frequency (Hz)"=w243, "Period (ms)"=w248, "Offset (V)"=w252, "Amplitude (V)"=w251, "Frequency"=w250, "Tri Repeats"=w249, "phase shift (ms)"=w248, "Pulses"=w248, "Matlab wave file"=path "", "Tri phase"=w247, "padding value"=w246) -> (w255:T18)
                            n3480 = Build Array(w255) -> (w254:T17)
                            n3481 = call "waveformparamsv2.vi"("command"="add AO", "add AO"=w254) -> ()  [unwired: 3 in, 3 out]
                          }
                        }
                      }
                    }
                  }
                  frame #5 {
                    n3482 = local read "addAO"() -> (w264:bool)
                    n3483 = case shown="True" w264 {
                      frame False {
                      }
                      frame True {
                        # "add waveform to waveform array; correct waveform lengths and plot"
                        n3484 = local read "Meastab"() -> (w268:enum32{"X-Y Image", "Linescan", "Timetrace"})
                        n3485 = local read "Build analog waveform tabs"() -> (w278:enum32{"Square", "Triangle", "Matlab"})
                        n3486 = case shown="\"Timetrace\"" w268 {
                          tunnel: [w286 w287] -> w267
                          frame "X-Y Image", Default {
                            n3487 = local read "Sampling rate"() -> (w286:dbl)
                          }
                          frame "Timetrace" {
                            n3488 = local read "srateAODOtt"() -> (w287:dbl)
                          }
                        }
                        n3489 = call "waveformparamsv2.vi"("command"="get last AO") -> ("last AO"=w280:T18)  [unwired: 4 in, 2 out]
                        n3490 = case shown="\"Matlab\"" w278 {
                          tunnel: w280 -> [w290 w292 w294]
                          tunnel: [w289 w291 w293] -> w279
                          frame "Square", Default {
                            n3491 = call "generateRampedSquareWave_fromAOparameters.vi"("AO params"=w290) -> ("Waveform"=w289:waveform(dbl))  [unwired: 1 out]
                          }
                          frame "Triangle" {
                            n3492 = call "generateTriWave_fromAOparameters.vi"("AO params"=w292) -> ("Waveform"=w291:waveform(dbl))  [unwired: 1 out]
                          }
                          frame "Matlab" {
                            n3493 = call "matlabAOwffromparam.vi"("Cluster"=w294) -> ("Waveform"=w293:waveform(dbl))  [unwired: 1 out]
                          }
                        }
                        n3494 = property on="refwf" class="Ring (strict)"() -> ("RingText.Text"=w271:string)  [unwired: 2 in, 2 out]
                        n3495 = call "waveformsAObuffer.vi"("command"="get") -> ("AO wf out"=w284:waveform(dbl)[])  [unwired: 1 in]
                        n3496 = Build Array (concatenate)(w284, w279) -> (w281:waveform(dbl)[])
                        n3497 = call "waveformsDObuffer.vi"("command"="get") -> ("DO wf out"=w276:digitalwaveform[])  [unwired: 1 in]
                        n3498 = call "correctwaveformsizetemp.vi"("new sampling frequency (Hz)"=w267, "start"=FALSE, "reference waveforms to"=w271, "Analog waveforms in"=w281, "stop"=FALSE, "Digital waveforms in"=w276) -> ("analog wf out"=w274:waveform(dbl)[], "Digital wf out"=w272:digitalwaveform[], "measpoints"=w269:i32)
                        n3499 = local write "Analog Lines Plot"(w274) -> ()
                        n3500 = call "GetNumCamFramesv2.vi"("Digital Waveform Graph"=w272) -> ("Numeric"=w273:i32)  [unwired: 10 in]
                        n3501 = local write "Digital Lines Plot"(w272) -> ()
                        n3502 = call "waveformsAObuffer.vi"("AO wf in"=w274, "command"="set") -> ()  [unwired: 1 out]
                        n3503 = call "waveformsDObuffer.vi"("DO wf in"=w272, "command"="set") -> ()  [unwired: 1 out]
                        n3504 = local write "Total Camera Frames"(w273) -> ()
                        n3505 = local read "wavdet"() -> (w270:bool)
                        n3506 = case shown="True" w270 {
                          tunnel: w269 -> [_ w288]
                          frame False {
                          }
                          frame True {
                            n3507 = local write "# of frames"(w288) -> ()
                          }
                        }
                      }
                    }
                  }
                  frame #6 {
                    w295 = FALSE ("addAO")
                    # "set signaling boolean to false"
                    n3508 = local read "finite samples"() -> (w296:bool)
                    n3509 = local read "continuous"() -> (w297:bool)
                    n3510 = local read "wavdet"() -> (w298:bool)
                    n3511 = call "2pparameters.vi"("command"="get") -> ("params out"=w301:T12)  [unwired: 1 in]
                    n3512 = Bundle By Name(cluster=w301, "finite"=w296, "cont"=w297, "wavdet"=w298) -> (w299:T12)
                    n3513 = local write "addAO"(w295) -> ()
                    n3514 = property on="Add AO wave" class="Bool (strict)"("Val(Sgnl)"=w295) -> ()  [unwired: 2 in, 2 out]
                    n3515 = call "2pparameters.vi"("Params in"=w299, "command"="set") -> ()  [unwired: 1 out]
                  }
                }
              }
            }
          }
          event "AO channels": Value Change {
            n3516 = event-data() -> ()  [unwired: 1 in, 6 out]
            n3517 = local read "AO channels"() -> (w303:u32)
            n3518 = call "2pparameters.vi"("command"="get") -> ("params out"=w305:T12)  [unwired: 1 in]
            n3519 = Unbundle By Name(w305) -> ("aAO"=w304:u32[])
            n3520 = Search 1D Array(1D array=w304, element=w303) -> (index of element=w307:i32)  [unwired: 1 in]
            n3521 = Equal?(x=w307, y=-1.0) -> (x = y?=w308:bool)
            n3522 = case shown="False" w308 {
              tunnel: w307 -> [w310 _]
              frame False {
                n3523 = call "waveformparamsv2.vi"("command"="get") -> ("Params out"=w317:T16)  [unwired: 4 in, 2 out]
                n3524 = Unbundle By Name(w317) -> ("AO parameters"=w316:T17)
                n3525 = Index Array(array=w316, index=w310) -> (element=w333:T18)
                n3526 = Unbundle By Name(w333) -> ("AOtab"=w314:dbl, "Repeats"=w332:dbl, "Cycles"=w331:dbl, "Start amplitude (V)"=w330:dbl, "Baseline (V)"=w329:dbl, "Step size (V)"=w328:dbl, "DC (%)"=w327:dbl, "Sampling frequency (Hz)"=w326:dbl, "Period (ms)"=w325:dbl, "Offset (V)"=w324:dbl, "Amplitude (V)"=w323:dbl, "Frequency"=w322:dbl, "Tri Repeats"=w321:dbl, "phase shift (ms)"=w320:dbl, "Pulses"=w319:dbl, "Tri phase"=w315:dbl, "padding value"=w311:dbl, "Matlab wave file"=w312:path)
                n3527 = To Unsigned Long Integer(number=w314) -> (unsigned 32bit integer=w313:u32)
                n3528 = local write "Build analog waveform tabs"(w313) -> ()
                n3529 = local write "Matlab waveform path"(w312) -> ()
                n3530 = local write "phase shift (ms)"(w320) -> ()
                n3531 = local write "Repeats"(w332) -> ()
                n3532 = local write "Cycles"(w331) -> ()
                n3533 = local write "Amplitude (V)"(w323) -> ()
                n3534 = local write "Matlab padding value"(w311) -> ()
                n3535 = local write "Tri padding value"(w311) -> ()
                n3536 = local write "Start amplitude (V)"(w330) -> ()
                n3537 = local write "Tri Phase (s)"(w315) -> ()
                n3538 = local write "Period (ms)"(w325) -> ()
                n3539 = local write "Tri Repeats"(w321) -> ()
                n3540 = local write "Offset (V)"(w324) -> ()
                n3541 = local write "Frequency"(w322) -> ()
                n3542 = local write "Pulses"(w319) -> ()
                n3543 = local write "padding value"(w311) -> ()
                n3544 = local write "Sampling rate \ncurrent wf"(w326) -> ()
                n3545 = local write "Baseline (V)"(w329) -> ()
                n3546 = local write "Step size (V)"(w328) -> ()
                n3547 = local write "DC (%)"(w327) -> ()
                "Numeric" <- w310
              }
              frame True {
              }
            }
          }
          event "Rem AO wave": Value Change {
            n3548 = event-data() -> ("NewVal"=w334:bool)  [unwired: 1 in, 5 out]
            n3549 = case shown="True" w334 {
              frame False {
              }
              frame True {
                n3550 = stacked-sequence {
                  seq-local: [_ _ w440 _ _ _ _] -> [_ _ _ _ w460 w463 _]
                  frame #0 {
                    n3551 = local read "Measurement"() -> (w335:T5)
                    n3552 = case shown="\"X-Y-t movie\", Default" w335 {
                      frame "X-Y-t movie", Default {
                        n3553 = local read "avpp"() -> (w356:i32)
                        n3554 = local read "Angle ref"() -> (w355:dbl)
                        n3555 = local read "ROI Type"() -> (w354:u16)
                        n3556 = local read "xpixels ref"() -> (w351:i32)
                        n3557 = local read "Vx-min ref"() -> (w350:dbl)
                        n3558 = local read "Vx-max ref"() -> (w349:dbl)
                        n3559 = local read "ypixels ref"() -> (w347:i32)
                        n3560 = local read "Vy-min ref"() -> (w348:dbl)
                        n3561 = local read "Vy-max ref"() -> (w344:dbl)
                        n3562 = local read "Sampling rate"() -> (w338:dbl)
                        n3563 = local read "finite samples"() -> (w339:bool)
                        n3564 = local read "continuous"() -> (w342:bool)
                        n3565 = local read "wavdet"() -> (w343:bool)
                        n3566 = local read "# of frames"() -> (w341:i32)
                        n3567 = local read "maxbufferAI"() -> (w340:i32)
                        n3568 = local read "Override AI buffer"() -> (w336:bool)
                        n3569 = call "2pparameters.vi"("command"="get") -> ("params out"=w353:T12)  [unwired: 1 in]
                        n3570 = Bundle By Name(cluster=w353, "type"="X-Y-t movie", "avpp"=w356, "Angle Img"=w355, "Xpixels Img"=w351, "Vx-min Img"=w350, "VX-max Img"=w349, "Ypixels Img"=w347, "Vy-min Img"=w348, "Vy-max Img"=w344, "srate"=w338, "srate Img"=w338, "finite"=w339, "cont"=w342, "wavdet"=w343, "measpoints"=w341, "maxbufferAI"=w340, "Drawing Mode"=w354, "Vz-reset"=0.0, "AIoverride"=w336) -> (w345:T12)
                        n3571 = call "2pparameters.vi"("Params in"=w345, "command"="set") -> ()  [unwired: 1 out]
                      }
                      frame "X-Y-Z stack" {
                        n3572 = call "2pparameters.vi"("command"="get") -> ("params out"=w360:T12)  [unwired: 1 in]
                        n3573 = Bundle By Name(cluster=w360, "type"="X-Y-Z stack") -> (w358:T12)
                        n3574 = call "2pparameters.vi"("Params in"=w358, "command"="set") -> ()  [unwired: 1 out]
                      }
                      frame "Lifetime (scan)" {
                        n3575 = call "2pparameters.vi"("command"="get") -> ("params out"=w365:T12)  [unwired: 1 in]
                        n3576 = Bundle By Name(cluster=w365, "type"="Lifetime (scan)") -> (w363:T12)
                        n3577 = call "2pparameters.vi"("Params in"=w363, "command"="set") -> ()  [unwired: 1 out]
                      }
                      frame "Lifetime (contour)" {
                        n3578 = local read "Vy-min draw"() -> (w375:dbl)
                        n3579 = local read "Vy-max draw"() -> (w374:dbl)
                        n3580 = local read "Vx-min draw"() -> (w377:dbl)
                        n3581 = local read "Vx-max draw"() -> (w376:dbl)
                        n3582 = local read "xpixels ref"() -> (w373:i32)
                        n3583 = local read "ypixels ref"() -> (w372:i32)
                        n3584 = local read "ROI Type"() -> (w371:u16)
                        n3585 = local read "srateAODOtt"() -> (w382:dbl)
                        n3586 = local read "# of frames"() -> (w387:i32)
                        n3587 = local read "refreshtime"() -> (w379:dbl)
                        n3588 = local read "Pel"() -> (w370:dbl)
                        n3589 = local read "bin"() -> (w385:dbl)
                        n3590 = local read "Override AI buffer"() -> (w368:bool)
                        n3591 = local read "finite samples"() -> (w394:bool)
                        n3592 = local read "srateAODOtt"() -> (w381:dbl)
                        n3593 = local read "srateAODOtt"() -> (w388:dbl)
                        n3594 = local read "continuous"() -> (w393:bool)
                        n3595 = local read "Angle ref"() -> (w378:dbl)
                        n3596 = local read "wavdet"() -> (w395:bool)
                        n3597 = local read "Vx-ref"() -> (w390:dbl)
                        n3598 = local read "Vy-ref"() -> (w392:dbl)
                        n3599 = local read "avpp"() -> (w391:i32)
                        n3600 = call "tt_timeandsamples.vi"("bin"=w385, "refreshtime"=w379, "srateAODOtt"=w382, "tot#ofsamples"=w387) -> ("refreshrate"=w383:dbl, "refreshbuffer"=w384:i32, "timetracecycles"=w389:i32)  [unwired: 5 in]
                        n3601 = local read "bin"() -> (w386:dbl)
                        n3602 = call "2pparameters.vi"("command"="get") -> ("params out"=w398:T12)  [unwired: 1 in]
                        n3603 = Bundle By Name(cluster=w398, "Drawing Mode"=w371, "measpoints"=w387, "tt_cycles"=w389, "refreshbuffer"=w384, "refreshrate"=w383, "Vx-ref"=w390, "Vy-ref"=w392, "srate"=w381, "finite"=w394, "cont"=w393, "wavdet"=w395, "avpp"=w391, "srateAODO"=w388, "bufferAI"=w384, "bin"=w386, "Angle Img"=w378, "Vxminref"=w377, "Vxmaxref"=w376, "Vyminref"=w375, "Vymaxref"=w374, "Xpixels Img"=w373, "Ypixels Img"=w372, "Pel"=w370, "Vz-reset"=0.0, "AIoverride"=w368, "type"="Lifetime (contour)") -> (w396:T12)
                        n3604 = Reciprocal(x=w383) -> (1/x=w380:dbl)
                        n3605 = local write "refreshtime"(w380) -> ()
                        n3606 = call "2pparameters.vi"("Params in"=w396, "command"="set") -> ()  [unwired: 1 out]
                      }
                      frame "X-Y-Z-t movie" {
                      }
                      frame "linescan" {
                      }
                      frame "Timetrace" {
                        n3607 = local read "Vy-min draw"() -> (w408:dbl)
                        n3608 = local read "Vy-max draw"() -> (w407:dbl)
                        n3609 = local read "Vx-min draw"() -> (w410:dbl)
                        n3610 = local read "Vx-max draw"() -> (w409:dbl)
                        n3611 = local read "xpixels ref"() -> (w406:i32)
                        n3612 = local read "ypixels ref"() -> (w405:i32)
                        n3613 = local read "ROI Type"() -> (w404:u16)
                        n3614 = local read "srateAODOtt"() -> (w415:dbl)
                        n3615 = local read "# of frames"() -> (w420:i32)
                        n3616 = local read "refreshtime"() -> (w412:dbl)
                        n3617 = local read "Pel"() -> (w403:dbl)
                        n3618 = local read "bin"() -> (w418:dbl)
                        n3619 = local read "Override AI buffer"() -> (w401:bool)
                        n3620 = local read "finite samples"() -> (w427:bool)
                        n3621 = local read "srateAODOtt"() -> (w414:dbl)
                        n3622 = local read "srateAODOtt"() -> (w421:dbl)
                        n3623 = local read "continuous"() -> (w426:bool)
                        n3624 = local read "Angle ref"() -> (w411:dbl)
                        n3625 = local read "wavdet"() -> (w428:bool)
                        n3626 = local read "Vx-ref"() -> (w423:dbl)
                        n3627 = local read "Vy-ref"() -> (w425:dbl)
                        n3628 = local read "avpp"() -> (w424:i32)
                        n3629 = call "tt_timeandsamples.vi"("bin"=w418, "refreshtime"=w412, "srateAODOtt"=w415, "tot#ofsamples"=w420) -> ("refreshrate"=w416:dbl, "refreshbuffer"=w417:i32, "timetracecycles"=w422:i32)  [unwired: 5 in]
                        n3630 = local read "bin"() -> (w419:dbl)
                        n3631 = call "2pparameters.vi"("command"="get") -> ("params out"=w431:T12)  [unwired: 1 in]
                        n3632 = Bundle By Name(cluster=w431, "Drawing Mode"=w404, "measpoints"=w420, "tt_cycles"=w422, "refreshbuffer"=w417, "refreshrate"=w416, "Vx-ref"=w423, "Vy-ref"=w425, "srate"=w414, "finite"=w427, "cont"=w426, "wavdet"=w428, "avpp"=w424, "srateAODO"=w421, "bufferAI"=w417, "bin"=w419, "Angle Img"=w411, "Vxminref"=w410, "Vxmaxref"=w409, "Vyminref"=w408, "Vymaxref"=w407, "Xpixels Img"=w406, "Ypixels Img"=w405, "Pel"=w403, "Vz-reset"=0.0, "AIoverride"=w401, "type"="Timetrace") -> (w429:T12)
                        n3633 = Reciprocal(x=w416) -> (1/x=w413:dbl)
                        n3634 = local write "refreshtime"(w413) -> ()
                        n3635 = call "2pparameters.vi"("Params in"=w429, "command"="set") -> ()  [unwired: 1 out]
                      }
                      frame "Lifetime (point)" {
                      }
                    }
                  }
                  frame #1 {
                    w434 = FALSE ("wavdet")
                    n3636 = call "2pparameters.vi"("command"="get") -> ("params out"=w438:T12)  [unwired: 1 in]
                    n3637 = Bundle By Name(cluster=w438, "finite"=w434, "cont"=w434, "wavdet"=TRUE) -> (w435:T12)
                    n3638 = call "2pparameters.vi"("Params in"=w435, "command"="set") -> ()  [unwired: 1 out]
                  }
                  frame #2 {
                    # "remove channel from numbers array"
                    n3639 = local read "AO channels"() -> (w445:u32)
                    n3640 = call "2pparameters.vi"("command"="get") -> ("params out"=w443:T12)  [unwired: 1 in]
                    n3641 = in-place {
                      in-place-border: w445 -> [w451]
                      in-place-border: [w448] -> w446
                      in-place-border: [w447] -> w440
                      n3642 = in-place-cluster #50(w443) -> ("aAO"=w450:u32[])
                      n3643 = call "remove channel from active arrayv2.vi"("line array in"=w450, "line to remove"=w451) -> ("line array out"=w449:u32[], "removal"=w448:bool, "index"=w447:i32)
                      n3644 = in-place-cluster #50("aAO"=w449) -> (w441:T12)
                    }
                    n3645 = local write "remAO"(w446) -> ()
                    n3646 = call "2pparameters.vi"("Params in"=w441, "command"="set") -> ()  [unwired: 1 out]
                  }
                  frame #3 {
                    n3647 = local read "remAO"() -> (w452:bool)
                    n3648 = case shown="True" w452 {
                      frame False {
                      }
                      frame True {
                        n3649 = call "Used AO lines.vi"() -> ("used AO names"=w456:string[], "used AO lines"=w458:tag[])  [unwired: 2 in]
                        n3650 = control-ref of="Analog Lines Plot"() -> (w457:refnum<vi>)
